vi "Streaming - Write Custom Cluster.vi"() -> ()   [LabVIEW 2020]
uses:
  Nominal Client/Nominal Client.lvclass/Nominal Client.ctl
  68d6fcb1-550e-49ab-bce3-21796ae30af0.vi
  Nominal Client/http.post.vi
  Nominal Client/private_data.set.vi
  68d6fcb1-550e-49ab-bce3-21796ae30af0.vi/8284acbc-2d4d-4b18-b492-8ff51a6e7e10.vi
  Nominal Client/trace.payload_received.vi
  Nominal Client/error.vi
  Nominal Client/trace.payload_sent.vi
  Nominal Client/create.authorization_header.vi
  nominal types/workspace/id.get.vi
  nominal types/workspace/rid.get.vi
  <vilib>/AdvancedString/1D String Array to Delimited String.vi
  Nominal Client/workspace.set.vi
  Nominal Client/trace.calling_method.vi
  Nominal Client/error.vi/859f8e04-e495-489b-b5b4-7ac163f56130.vi
  <vilib>/JDP Science/JDP Science Common Utilities/Trim Whitespace__JDP.vi
  Nominal Client/api_token.get.vi
  <vilib>/Utility/file.llb/Application Directory.vi
  <vilib>/Utility/error.llb/Error Cluster From Error Code.vi
  Nominal Client/format endpoint termination.vi
  submodules/reqwest-labview/lv-src/reqwest/create.vi
  Nominal Client/workspace_cache.get_from_rid.vi
  Nominal Client/workspace_cache.get.vi
  Nominal Client/Palette Items/who_am_i.vi
  stream_custom_cluster/to json.vi
  <vilib>/Utility/libraryn.llb/Get File Extension.vi
  Nominal Client/log_file.write.vi
  submodules/reqwest-labview/lv-src/reqwest/post.vi
  <vilib>/JDP Science/JSONtext/Get all Object Items.vi
  <vilib>/JDP Science/JSONtext/JSON text to Variant.vi
  User/User.lvclass
  Nominal Client/Nominal Client.lvclass
  nominal types/workspace/workspace.lvclass
  submodules/reqwest-labview/lv-src/reqwest/reqwest.lvclass
  <vilib>/JDP Science/JSONtext/LVClass Serializer/JSONtext LVClass Serializer.lvclass
  stream_custom_cluster/stream_custom_cluster.lvclass
panel:
  in  "API Token (string or path)":string
  in  "Data Source RID":string
  out "Consumer Stopped":bool
  in  "Data Cluster":T1 {"asdfHorizontal Pointer Slide" scale=0.0..10.0}
  in  "Stop":bool
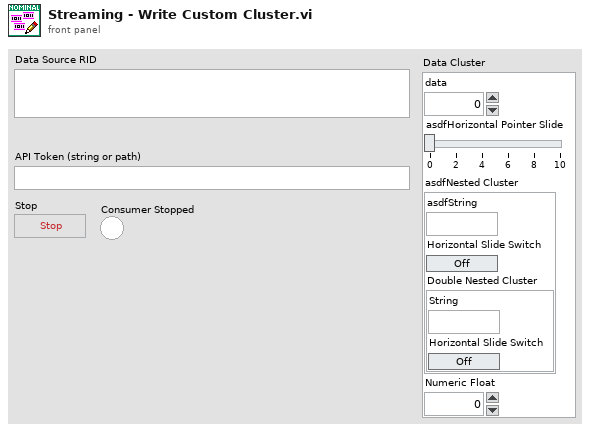
[diagram p1: front panel]
types:
  T1 = cluster{"data":i32, "asdfHorizontal Pointer Slide":dbl, "asdfNested Cluster":cluster{"asdfString":string, "Horizontal Slide Switch":bool, "Double Nested Cluster":cluster{"String":string, "Horizontal Slide Switch":bool}}, "Numeric Float":dbl}
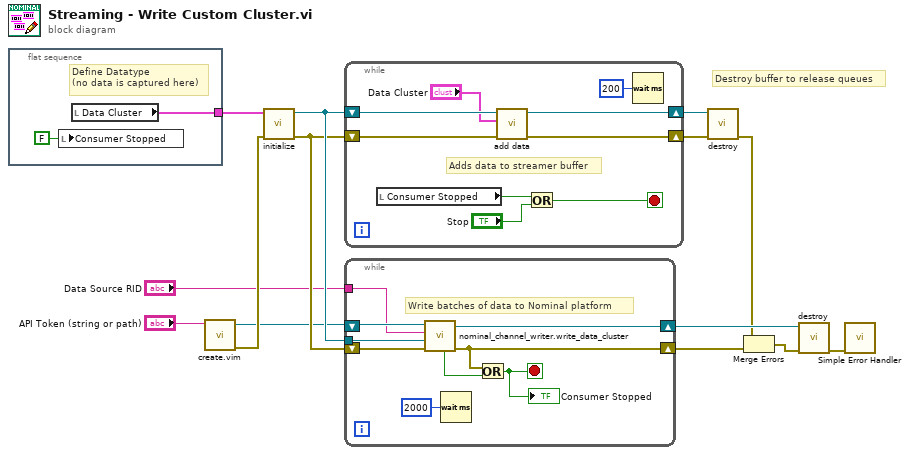
[diagram p0: block diagram]
diagram:
  # "Destroy buffer to release queues"
  n1 = flat-sequence {
    tunnel: [w16] -> w10
    frame #0 {
      # "Define Datatype\n(no data is captured here)"
      n2 = local write "Consumer Stopped"(FALSE ("Consumer Stopped")) -> ()
      n3 = local read "Data Cluster"() -> (w16:T1)
    }
  }
  n4 = call "create.vim"("API Token (string or path)"="API Token (string or path)") -> ("error out"=w9:errorcluster, "Nominal Client"=w1:refnum<class "Nominal Client.lvclass">)  [unwired: 8 in, 1 out]
  n5 = call "initialize.vi"("error in"=w9, "Data Cluster"=w10) -> ("error out"=w12:errorcluster, "stream custom cluster"=w13:refnum<class "stream_custom_cluster.lvclass">)  [unwired: 8 in]
  n6 = while {
    shift-right: [w21] -> w11
    shift-left: w12 -> [w22]
    shift-right: [w24] -> w14
    shift-left: w13 -> [w25]
    stop <- w17 stop-if-true
    # "Adds data to streamer buffer"
    n7 = local read "Consumer Stopped"() -> (w19:bool)
    n8 = call "add data.vi"("error in"=w22, "Data Cluster"="Data Cluster", "stream custom cluster in"=w25) -> ("error out"=w21:errorcluster, "stream custom cluster out"=w24:refnum<class "stream_custom_cluster.lvclass">)  [unwired: 7 in]
    n9 = Or(x=w19, y="Stop") -> (x .or. y?=w17:bool)
    n10 = Wait (ms)(milliseconds to wait=u32 200) -> ()  [unwired: 1 out]
  }
  n11 = while {
    tunnel: w13 -> [w33]
    shift-right: [w30] -> w8
    shift-left: w1 -> [w31]
    tunnel: "Data Source RID" -> [w29]
    shift-right: [w28] -> w4
    shift-left: w12 -> [w32]
    stop <- w26 stop-if-true
    # "Write batches of data to Nominal platform"
    n12 = call "nominal_channel_writer.write_data_cluster.vi"("error in"=w32, "Custom Cluster Streamer"=w33, "Data Source RID"=w29, "Nominal Client in"=w31) -> ("error out"=w28:errorcluster, "Nominal Client out"=w30:refnum<class "Nominal Client.lvclass">, "Terminated"=w27:bool)  [unwired: 5 in]
    n13 = Wait (ms)(milliseconds to wait=u32 2000) -> ()  [unwired: 1 out]
    n14 = Or(x=w28, y=w27) -> (x .or. y?=w26:bool)
    "Consumer Stopped" <- w26
  }
  n15 = call "destroy.vi"("error in"=w11, "stream custom cluster"=w14) -> ("error out"=w5:errorcluster)  [unwired: 9 in]
  n16 = Merge Errors(w5, w4) -> (w3:errorcluster)
  n17 = call "destroy.vi"("error in"=w3, "Nominal Client"=w8) -> ("error out"=w2:errorcluster)  [unwired: 9 in]
  n18 = call <vilib>:"Simple Error Handler.vi"("error in (no error)"=w2) -> ()  [unwired: 4 in, 5 out]
